vi "UV Disinfectant code.vi"() -> ()   [LabVIEW 2019]
uses:
  <vilib>/MakerHub/LINX/Public/Peripherals/Digital/Digital Read 1 Chan.vi
  <vilib>/MakerHub/LINX/Public/Peripherals/Digital/Digital Write 1 Chan.vi
  <vilib>/MakerHub/LINX/Public/Peripherals/Digital/Digital Read N Chans.vi
  <vilib>/MakerHub/LINX/Public/Peripherals/Digital/Digital Write N Chans.vi
  <vilib>/MakerHub/LINX/Private/Local IO/LinxDigitalRead.vi
  <vilib>/MakerHub/LINX/Public/Utilities/Check Channel.vi
  <vilib>/MakerHub/LINX/Private/Local IO/LinxDigitalWrite.vi
  <vilib>/MakerHub/LINX/Public/Utilities/Open Serial.vi
  <vilib>/MakerHub/LINX/Private/Utilties/Generate Error.vi
  <vilib>/ErrorRing/Error Ring.xnode
  <vilib>/MakerHub/LINX/LMH-LINX.lvlib
panel:
  out "Time for which lamp stays ON":dbl caption="Elapsed Time (s)"
  out "UV Lamp":bool
  in  "stop":bool
  out "REED Input":bool
  in  "Serial Port":refnum<visa-resource-name>="N/A"
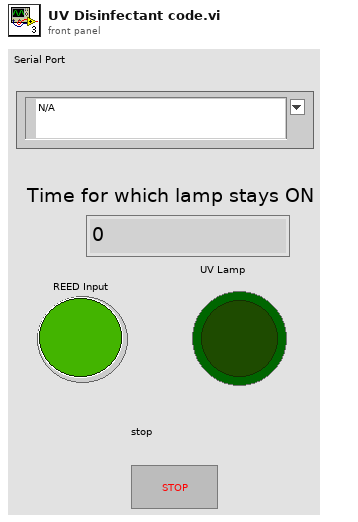
[diagram p1: front panel]
types:
  T1 = typedef "LMH-LINX.lvlib/LINX Ref.ctl" = cluster{"IO":T2, "Interface":T3, "LINX Device Config":T4}
  T2 = typedef "LMH-LINX.lvlib/Platform.ctl" = enum16{"Remote", "Local"}
  T3 = typedef "LMH-LINX.lvlib/Interface.ctl" = enum16{"Serial", "TCP"}
  T4 = typedef "LMH-LINX.lvlib/Device.lvlib/LINX Device Config.ctl" = cluster{"Interface":T3, "COM Port":refnum<visa-resource-name>, "TCP Configuration":T5, "Device Family":u8, "Device ID":u8, "Device Name":string, "TCP Ref":refnum<k5>, "Channels":T6}
  T5 = typedef "LMH-LINX.lvlib/Device.lvlib/TCP Config.ctl" = cluster{"IP Address":string, "Port":u16}
  T6 = typedef "LMH-LINX.lvlib/Channels.ctl" = cluster{"DI":u8[], "DO":u8[], "AI":u8[], "AO":u8[], "PWM":u8[], "QE":u8[], "UART":u8[], "I2C 2":u8[], "SPI":u8[], "CAN":u8[], "Servo":u8[], "AI Ref (V)":dbl, "AI Resolution (Bits)":u8, "AO Ref (V)":dbl, "AO Resolution (Bits)":u8}
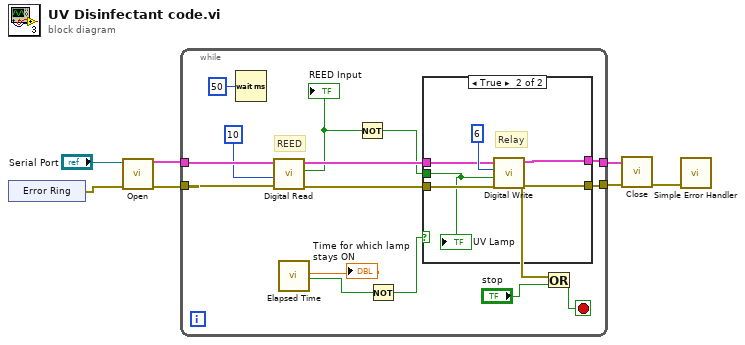
[diagram p0: block diagram]
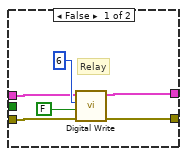
[diagram p2: hidden frame]
diagram:
  n1 = xnode ("Error Ring")() -> ("error out"=w6:errorcluster)
  n2 = call-poly <vilib>:"Open.vi"("Error In"=w6, "Serial Port"="Serial Port") -> ("Error Out"=w4:errorcluster, "LINX Resource"=w5:T1)  [unwired: 7 in, 1 out]
  n3 = while {
    tunnel: w5 -> [w22]
    tunnel: w4 -> [w21]
    tunnel: [w19] -> w3
    tunnel: [w15] -> w2
    stop <- w16 stop-if-true
    # "REED"
    n4 = Wait (ms)(milliseconds to wait=u32 50) -> ()  [unwired: 1 out]
    n5 = call-poly <vilib>:"Digital Read.vi"("Error In"=w21, "DI Channel"=u8 10, "LINX Resource"=w22) -> ("Error Out"=w13:errorcluster, "DI Value"=w8:bool, "LINX Resource"=w14:T1)  [unwired: 6 in]
    "REED Input" <- w8
    n6 = call "Elapsed Time"() -> ("Elapsed Time (s)"=→"Time for which lamp stays ON":dbl, "Time has Elapsed"=w12:bool)  [unwired: 12 in, 6 out]
    n7 = Not(x=w8) -> (.not. x?=w9:bool)
    n8 = Not(x=w12) -> (.not. x?=w11:bool)
    n9 = case shown="True" w11 {
      tunnel: [w25 w33] -> w19
      tunnel: [w24 w32] -> w15
      tunnel: w14 -> [w27 w31]
      tunnel: w13 -> [w26 w30]
      tunnel: w9 -> [_ w29]
      frame False {
        # "Relay"
        n10 = call-poly <vilib>:"Digital Write.vi"("Error In"=w26, "Output Value"=FALSE, "DO Channel"=u8 6, "LINX Resource"=w27) -> ("Error Out"=w24:errorcluster, "LINX Resource"=w25:T1)  [unwired: 6 in]
      }
      frame True {
        # "Relay"
        n11 = call-poly <vilib>:"Digital Write.vi"("Error In"=w30, "Output Value"=w29, "DO Channel"=u8 6, "LINX Resource"=w31) -> ("Error Out"=w32:errorcluster, "LINX Resource"=w33:T1)  [unwired: 6 in]
        "UV Lamp" <- w29
      }
    }
    n12 = Or(x=w15, y="stop") -> (x .or. y?=w16:bool)
  }
  n13 = call <vilib>:"Close.vi"("Error In"=w2, "LINX Resource"=w3) -> ("Error Out"=w1:errorcluster)  [unwired: 9 in]
  n14 = call <vilib>:"Simple Error Handler.vi"("error in (no error)"=w1) -> ()  [unwired: 4 in, 5 out]
